vi "Read Digital All Pins.vi"(8 "error in (no error)":errorcluster, 11 "Chip Address (A2 A1 A0)":T2 max=7) -> (0 "error out":errorcluster, 3 "SPI Command":T1)   [LabVIEW 2014, in "SLSC configuration Shared.lvlib"]
doc: "Reads the GPIO state of all pins."
uses:
  SLSC configuration Shared.lvlib
  Chip Address.ctl
  SPI Command.ctl
  OPCODE.ctl
  IOCON BANK 0 Reg Addresses.ctl
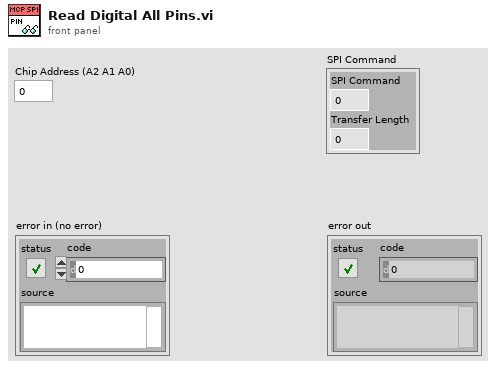
[diagram p1: front panel]
types:
  T1 = typedef "SLSC configuration Shared.lvlib/SPI Command.ctl" = cluster{"SPI Command":u32, "Transfer Length":u8}
  T2 = typedef "SLSC configuration Shared.lvlib/Chip Address.ctl" = u8
  T3 = typedef "SLSC configuration Shared.lvlib/IOCON BANK 0 Reg Addresses.ctl" = enum8{"IODIRA", "IODIRB", "IPOLA", "IPOLB", "GPINTENA", "GPINTENB", "DEFVALA", "DEFVALB", "INTCONA", "INTCONB", "IOCONA", "IOCONB", "GPPUA", "GPPUB", "INTFA", "INTFB", "INTCAPA", "INTCAPB", "GPIOA", "GPIOB", "OLATA", "OLATB"}
  T4 = typedef "SLSC configuration Shared.lvlib/OPCODE.ctl" = u8
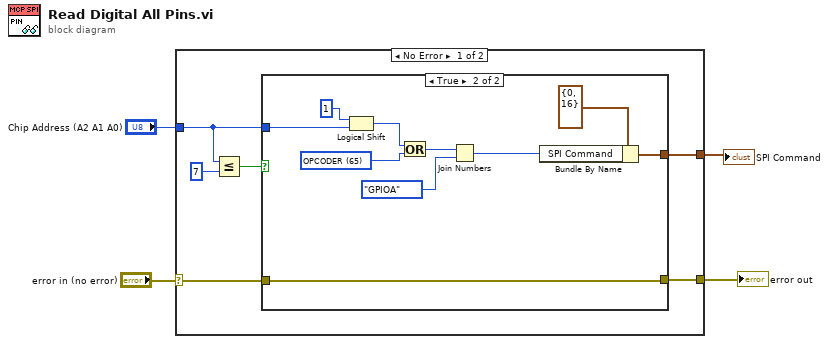
[diagram p0: block diagram]
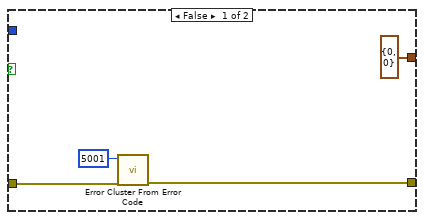
[diagram p2: hidden frame]
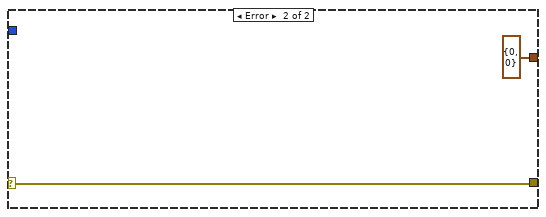
[diagram p3: hidden frame]
diagram:
  n1 = case shown="No Error" "error in (no error)" {
    selector: "error in (no error)" -> [w7 w26]
    tunnel: "Chip Address (A2 A1 A0)" -> [w10 _]
    tunnel: [w6 w26] -> w2
    tunnel: [w5 T1 {"SPI Command"=0, "Transfer Length"=0} ("SPI Command")] -> w1
    frame No Error {
      n2 = Less Or Equal?(x=w10, y=T2 7) -> (x <= y?=w9:bool)
      n3 = case shown="True" w9 {
        tunnel: w10 -> [_ w24]
        tunnel: w7 -> [w13 w18]
        tunnel: [w12 w18] -> w6
        tunnel: [T1 {"SPI Command"=0, "Transfer Length"=0} ("SPI Command") w15] -> w5
        frame False {
          n4 = call <vilib>:"Error Cluster From Error Code.vi"("error in (no error)"=w13, "error code (0)"=5001) -> ("error out"=w12:errorcluster)  [unwired: 7 in]
        }
        frame True {
          w21 = T4 65 items=["OPCODEW"=64, "OPCODER"=65, "ADDR_ENABLE"=8] ("OPCODE")
          n5 = Logical Shift(y=u8 1, x=w24) -> (x << y=w22:T2)
          n6 = Or(x=w22, y=w21) -> (x .or. y?=w20:T2)
          n7 = Join Numbers(hi=w20, lo=IOCON_BANK_0_Reg_Addresses."GPIOA" ("IOCON.BANK = 0 Reg Addresses")) -> ((hi.lo)=w16:u16)
          n8 = Bundle By Name(cluster=T1 {"SPI Command"=0, "Transfer Length"=16} ("SPI Command"), "SPI Command"=w16) -> (w15:T1)
        }
      }
    }
    frame Error {
    }
  }
  "error out" <- w2
  "SPI Command" <- w1
